vi "Tag Watchlist UI.vi"(6 "Shutdown Event":refnum<user-event>) -> ()   [LabVIEW 2020, in "Tag Watchlist.lvlib"]
doc: "Tag Watchlist window can view and modify any existing Tag.\n\nUse the Watchlist launcher to run this VI in your application."
uses:
  Tag Watchlist.lvlib
  Tag/Tag.lvclass
  Tag/Tag.lvclass/Tag.ctl
  Tag/Read Name.vi
  Tag/Read Type.vi
  Tag/Read Description.vi
  Tag/Read Units.vi
  Tag/Read Stale.vi
  Tag/Read Value.vi
  Tag/Read Timestamp.vi
  Core/Tag Lookup_By Name.vi
  <vilib>/Utility/Data Type/Get Type Information.vi
  <vilib>/JDP Science/JSONtext/Variant to JSON Text.vi
  Tag Engine.lvlib
panel:
  in  "Watchlist":i32(listbox)
  in  "Tag List":i32(listbox)
  in  "Filter":string
  # "Tag Engine Debug Watchlist Window"
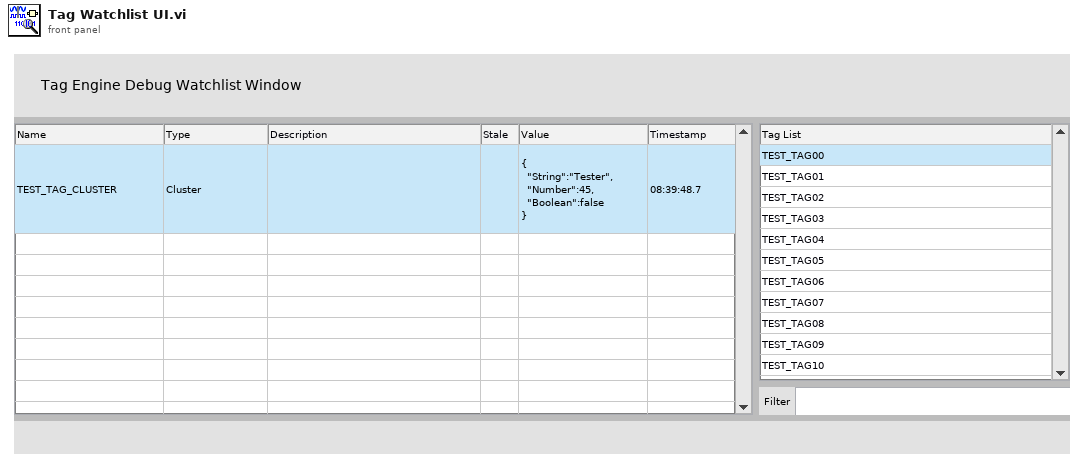
[diagram p1: front panel]
types:
  T1 = typedef "LVPoint32TypeDef.ctl" = cluster{"Horizontal":i32, "Vertical":i32}
  T2 = typedef "NI_Data Type.lvlib/Data Type.ctl" = enum8{"Invalid Type", "Void", "I8", "I16", "I32", "I64", "U8", "U16", "U32", "U64", "Single Float", "Double Float", "Extended Float", "Single Complex", "Double Complex", "Extended Complex", "Enum U8", "Enum U16", "Enum U32", "Enum U64", "Single Float With Unit", "Double Float With Unit", "Extended Float With Unit", "Single Complex with Unit", "Double Complex with Unit", "Extended Complex with Unit", "Boolean", "String", "Path", "Picture", "Tag", "Array", "Cluster", "Variant", "LV Variant", "Waveform", "Timestamp", "Digital Waveform", "Digital Data", "ExpressData", "Refnum", "External Data", "VI", "Poly VI", "LabVIEW Class Instance", "Fixed Point", "Set Collection", "Map Collection"}
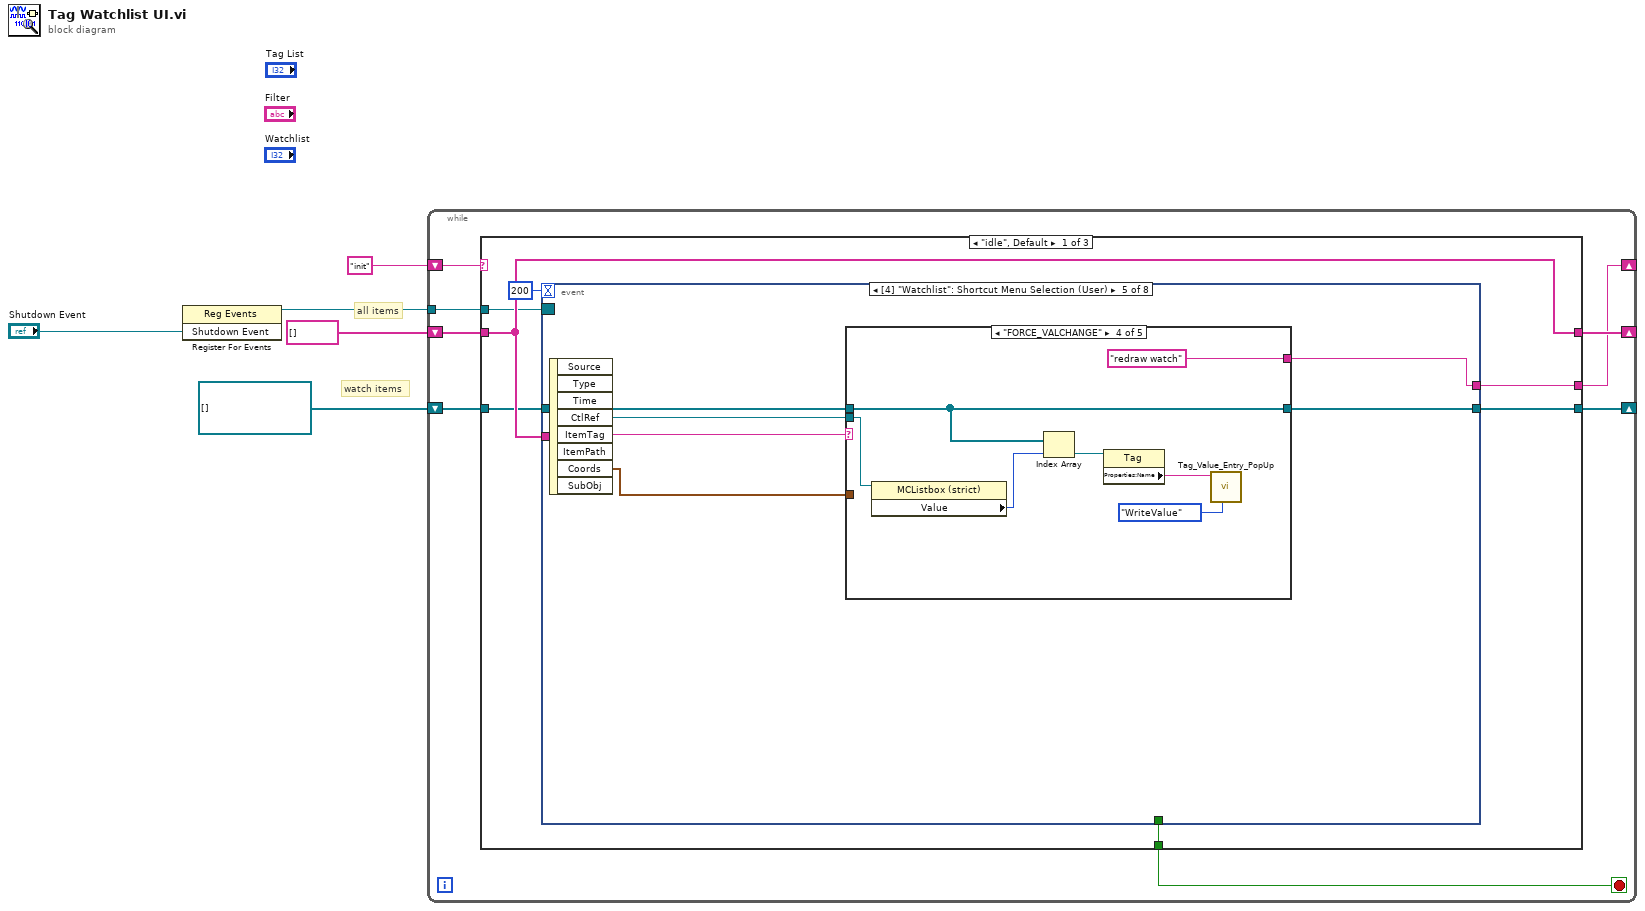
[diagram p0: block diagram]
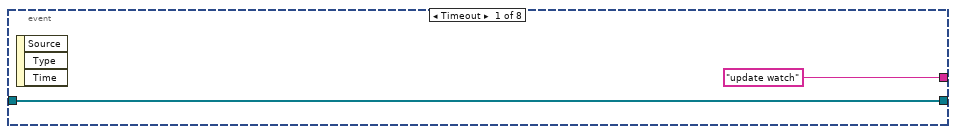
[diagram p2: hidden frame]
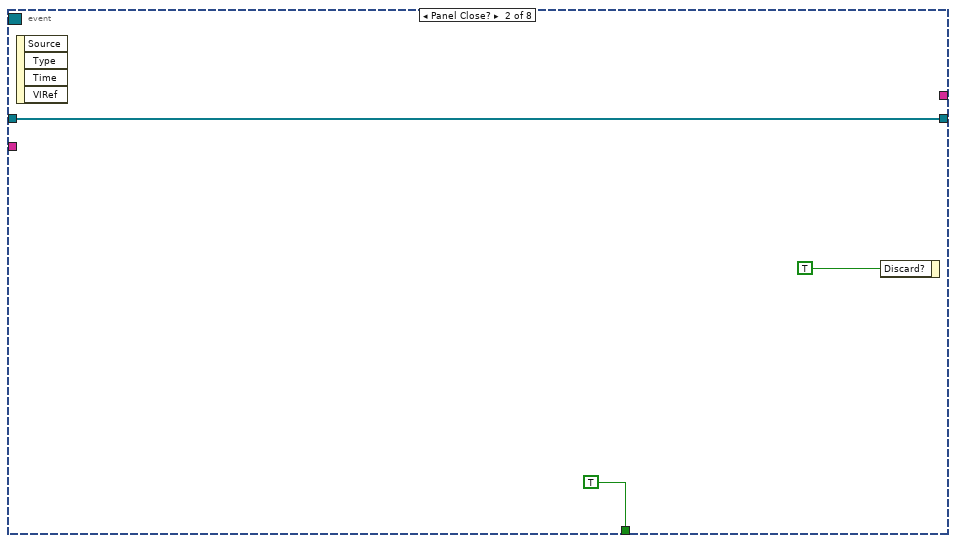
[diagram p3: hidden frame]
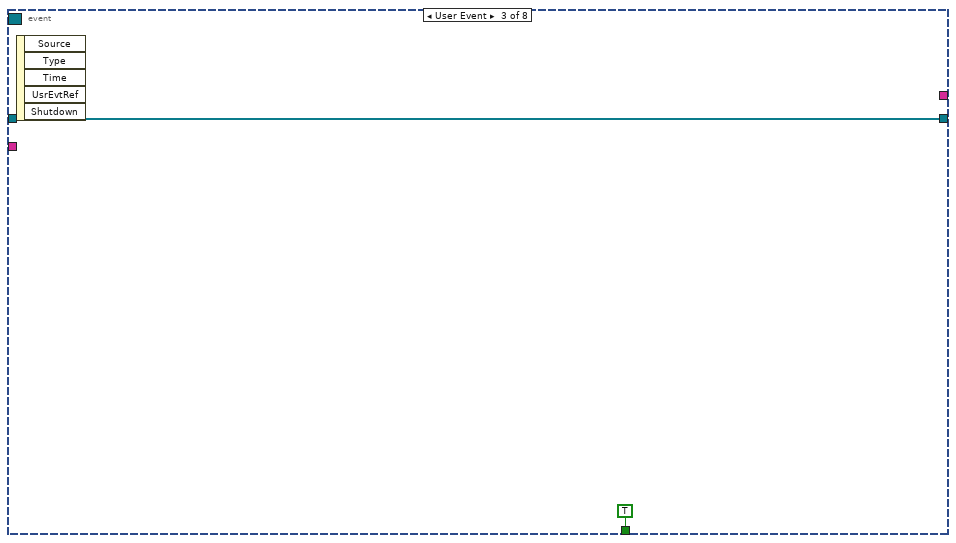
[diagram p4: hidden frame]
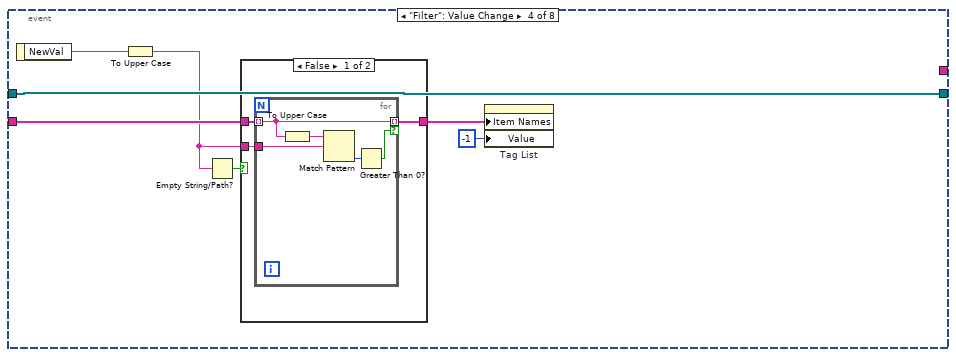
[diagram p5: hidden frame]
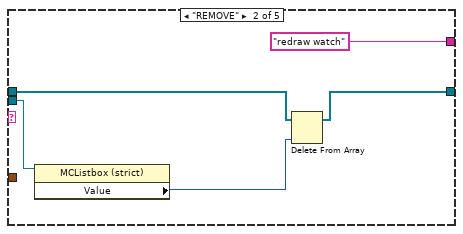
[diagram p8: hidden frame]
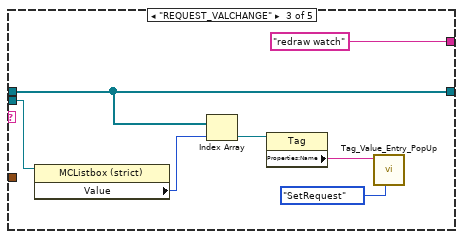
[diagram p9: hidden frame]
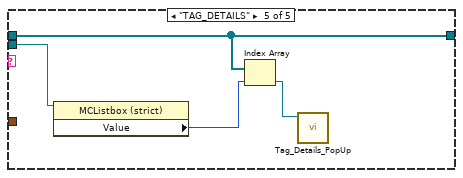
[diagram p10: hidden frame]
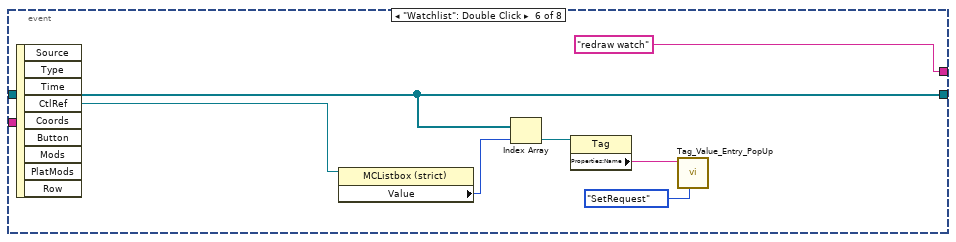
[diagram p11: hidden frame]
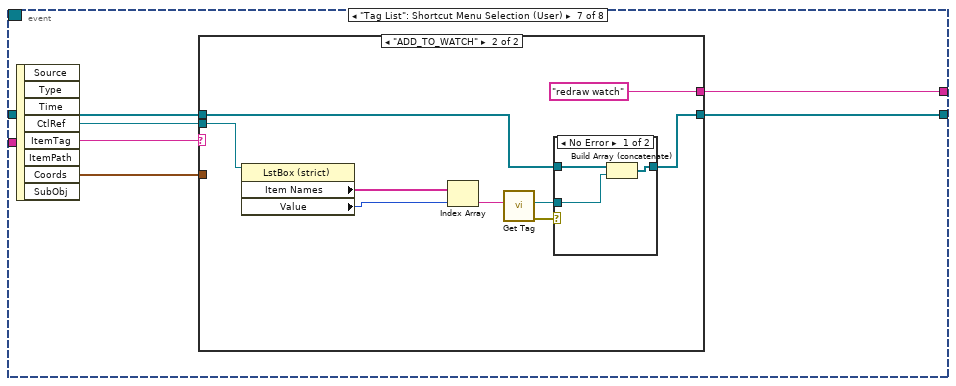
[diagram p12: hidden frame]
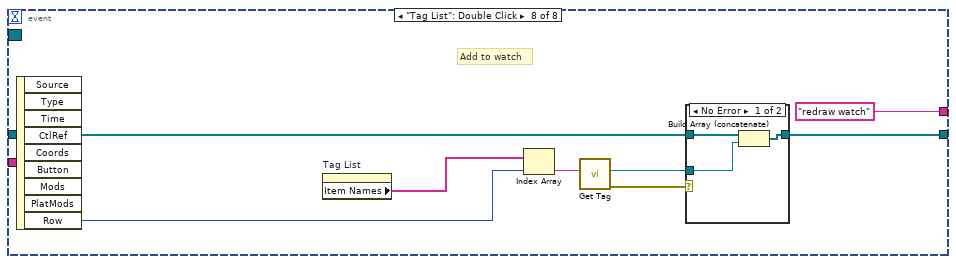
[diagram p15: hidden frame]
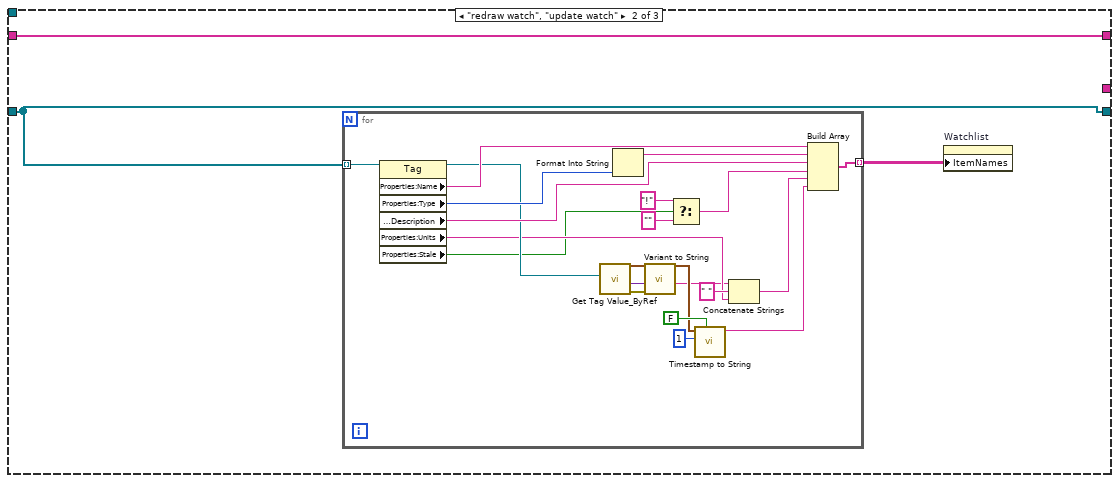
[diagram p17: hidden frame]
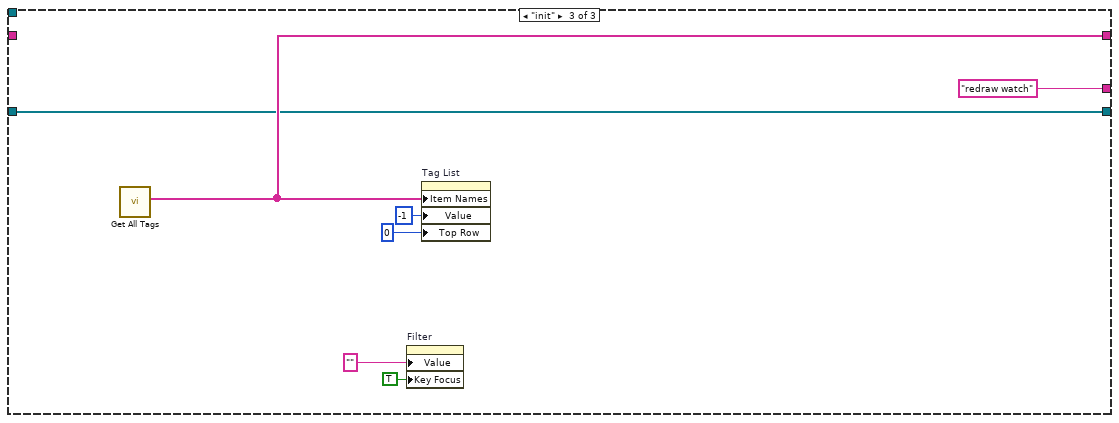
[diagram p18: hidden frame]
diagram:
  # "watch items"
  # "all items"
  n1 = register-events("Shutdown Event") -> (reference out=w2:refnum<event-registration>)  [unwired: 2 in, 1 out]
  n2 = while {
    shift-right: [w7] -> _
    shift-left: "init" -> [w13]
    shift-right: [w12] -> _
    shift-left: string[] [] ("Tag Names") -> [w11]
    shift-right: [w8] -> _
    shift-left: refnum<data-value>[] [] ("Item ref out") -> [w9]
    tunnel: w2 -> [w6]
    stop <- w10 stop-if-true
    n3 = case shown="\"idle\", Default" w13 {
      tunnel: [w19 w115 w143] -> w12
      tunnel: w11 -> [w19 w115 _]
      tunnel: [w20 _ _] -> w10
      tunnel: w9 -> [w18 w114 w142]
      tunnel: [w17 w114 w142] -> w8
      tunnel: [w15 _ "redraw watch"] -> w7
      tunnel: w6 -> [w14 _ _]
      frame "idle", Default {
        n4 = event shown="[4] \"Watchlist\": Shortcut Menu Selection (User)" {
          selector: w14 -> [_ _ _ _ _ _ _ _]
          dyn-events: _ -> [_ _ _ _ _ _ _ _]
          timeout: 200 -> [_ _ _ _ _ _ _ _]
          tunnel: [_ TRUE TRUE _ _ _ _ _] -> w20
          tunnel: w19 -> [_ _ _ w34 _ _ _ _]
          tunnel: w18 -> [w22 w23 w26 w31 w47 w80 w82 w108]
          tunnel: [w22 w23 w26 w31 w46 w80 w81 w107] -> w17
          tunnel: ["update watch" _ _ _ w45 "redraw watch" w85 "redraw watch"] -> w15
          event Timeout {
            n5 = event-data() -> ()  [unwired: 1 in, 3 out]
          }
          event Panel Close? {
            n6 = event-data() -> ()  [unwired: 1 in, 4 out]
            n7 = event-data("Discard?"=TRUE) -> ()  [unwired: 1 in, 1 out]
          }
          event User Event {
            n8 = event-data() -> ()  [unwired: 1 in, 5 out]
          }
          event "Filter": Value Change {
            n9 = event-data() -> ("NewVal"=w29:string)  [unwired: 1 in]
            n10 = To Upper Case(1:w29) -> (0:w28:string)
            n11 = Empty String/Path?(string/path=w28) -> (empty?=w30:bool)
            n12 = case shown="False" w30 {
              tunnel: w34 -> [w37 w43]
              tunnel: [w36 w43] -> w33
              tunnel: w28 -> [w35 _]
              frame False {
                n13 = for {
                  tunnel: w35 -> [w42]
                  tunnel: w37 -> [w39] mode=indexing
                  tunnel: [w39] -> w36 mode=indexing if=w40
                  n14 = To Upper Case(1:w39) -> (0:w38:string)
                  n15 = Match Pattern(string=w38, regular expression=w42) -> (offset past match=w41:i32)  [unwired: 1 in, 3 out]
                  n16 = Greater Than 0?(x=w41) -> (x > 0?=w40:bool)
                }
              }
              frame True {
              }
            }
            n17 = property on="Tag List" class="LstBox (strict)"("Item Names"=w33, "Value"=-1 ("Tag List")) -> ()  [unwired: 2 in, 2 out]
          }
          event "Watchlist": Shortcut Menu Selection (User) {
            n18 = event-data() -> ("CtlRef"=w44:refnum<vi>, "ItemTag"=w49:string, "Coords"=w48:T1)  [unwired: 1 in, 5 out]
            n19 = case shown="\"FORCE_VALCHANGE\"" w49 {
              tunnel: w48 -> [_ _ _ _ _]
              tunnel: w47 -> [w50 w55 w58 w65 w72]
              tunnel: [w50 w54 w58 w65 w72] -> w46
              tunnel: [_ "redraw watch" "redraw watch" "redraw watch" _] -> w45
              tunnel: w44 -> [_ w52 w61 w68 w73]
              frame Default {
              }
              frame "REMOVE" {
                n20 = property class="MCListbox (strict)"(reference=w52) -> ("Value"=w51:i32)  [unwired: 1 in, 2 out]
                n21 = Delete From Array(array=w55, index=w51) -> (array with subset deleted=w54:refnum<data-value>[])  [unwired: 1 in, 1 out]
              }
              frame "REQUEST_VALCHANGE" {
                n22 = property class="MCListbox (strict)"(reference=w61) -> ("Value"=w60:i32)  [unwired: 1 in, 2 out]
                n23 = Index Array(array=w58, index=w60) -> (element=w59:refnum<data-value>)
                n24 = property class="Tag"(reference=w59) -> ("Properties:Name"=w57:string)  [unwired: 1 in, 2 out]
                n25 = call "Tag_Value_Entry_PopUp.vi"("Write Type"=enum16{"SetRequest", "WriteValue"}."SetRequest", "Tag Name"=w57) -> ()  [unwired: 6 in, 4 out]
              }
              frame "FORCE_VALCHANGE" {
                n26 = property class="MCListbox (strict)"(reference=w68) -> ("Value"=w67:i32)  [unwired: 1 in, 2 out]
                n27 = Index Array(array=w65, index=w67) -> (element=w66:refnum<data-value>)
                n28 = property class="Tag"(reference=w66) -> ("Properties:Name"=w64:string)  [unwired: 1 in, 2 out]
                n29 = call "Tag_Value_Entry_PopUp.vi"("Write Type"=enum16{"SetRequest", "WriteValue"}."WriteValue", "Tag Name"=w64) -> ()  [unwired: 6 in, 4 out]
              }
              frame "TAG_DETAILS" {
                n30 = property class="MCListbox (strict)"(reference=w73) -> ("Value"=w71:i32)  [unwired: 1 in, 2 out]
                n31 = Index Array(array=w72, index=w71) -> (element=w70:refnum<data-value>)
                n32 = call "Tag_Details_PopUp.vi"("Tag Ref in"=w70) -> ()  [unwired: 10 in, 1 out]
              }
            }
          }
          event "Watchlist": Double Click {
            n33 = event-data() -> ("CtlRef"=w78:refnum<vi>)  [unwired: 1 in, 8 out]
            n34 = property class="MCListbox (strict)"(reference=w78) -> ("Value"=w77:i32)  [unwired: 1 in, 2 out]
            n35 = Index Array(array=w80, index=w77) -> (element=w76:refnum<data-value>)
            n36 = property class="Tag"(reference=w76) -> ("Properties:Name"=w75:string)  [unwired: 1 in, 2 out]
            n37 = call "Tag_Value_Entry_PopUp.vi"("Write Type"=enum16{"SetRequest", "WriteValue"}."SetRequest", "Tag Name"=w75) -> ()  [unwired: 6 in, 4 out]
          }
          event "Tag List": Shortcut Menu Selection (User) {
            n38 = event-data() -> ("CtlRef"=w84:refnum<vi>, "ItemTag"=w86:string, "Coords"=w83:T1)  [unwired: 1 in, 5 out]
            n39 = case shown="\"ADD_TO_WATCH\"" w86 {
              tunnel: [_ "redraw watch"] -> w85
              tunnel: w84 -> [_ w91]
              tunnel: w83 -> [_ _]
              tunnel: w82 -> [w87 w90]
              tunnel: [w87 w89] -> w81
              frame Default {
              }
              frame "ADD_TO_WATCH" {
                n40 = property on="Property Node" class="LstBox (strict)"(reference=w91) -> ("Item Names"=w95:string[], "Value"=w88:i32)  [unwired: 1 in, 2 out]
                n41 = Index Array(array=w95, index=w88) -> (element=w94:string)
                n42 = call "Get Tag.vi"("Name"=w94) -> ("error out"=w93:errorcluster, "Tag Ref out"=w92:refnum<data-value>)  [unwired: 8 in, 1 out]
                n43 = case shown="No Error" w93 {
                  tunnel: w90 -> [w99 w100]
                  tunnel: w92 -> [w98 _]
                  tunnel: [w97 w100] -> w89
                  frame No Error {
                    n44 = Build Array (concatenate)(w99, w98) -> (w97:refnum<data-value>[])
                  }
                  frame Error {
                  }
                }
              }
            }
          }
          event "Tag List": Double Click {
            # "Add to watch"
            n45 = event-data() -> ("Row"=w102:i32)  [unwired: 1 in, 8 out]
            n46 = property on="Tag List" class="LstBox (strict)"() -> ("Item Names"=w106:string[])  [unwired: 2 in, 2 out]
            n47 = Index Array(array=w106, index=w102) -> (element=w105:string)
            n48 = call "Get Tag.vi"("Name"=w105) -> ("error out"=w104:errorcluster, "Tag Ref out"=w103:refnum<data-value>)  [unwired: 8 in, 1 out]
            n49 = case shown="No Error" w104 {
              tunnel: w108 -> [w111 w112]
              tunnel: w103 -> [w110 _]
              tunnel: [w109 w112] -> w107
              frame No Error {
                n50 = Build Array (concatenate)(w111, w110) -> (w109:refnum<data-value>[])
              }
              frame Error {
              }
            }
          }
        }
      }
      frame "redraw watch", "update watch" {
        n51 = for {
          tunnel: w114 -> [w136] mode=indexing
          tunnel: [w128] -> w113 mode=indexing
          n52 = property class="Tag"(reference=w136) -> (reference out=w127:refnum<data-value>, "Properties:Name"=w134:string, "Properties:Type"=w135:T2, "Properties:Description"=w132:string, "Properties:Units"=w124:string, "Properties:Stale"=w122:bool)  [unwired: 1 in, 1 out]
          n53 = call "Get Tag Value_ByRef.vi"("Tag Ref in"=w127) -> ("error out"=w118:errorcluster, "Value"=w117:variant, "Timestamp"=w126:timestamp)  [unwired: 7 in, 1 out]
          n54 = Format Into String(w135) -> (resulting string=w133:string)  [unwired: 3 in, 1 out]
          n55 = call "Variant to String.vi"("error in"=w118, "Variant Value"=w117) -> ("String Value"=w116:string)  [unwired: 8 in, 1 out]
          n56 = Select(t="!", s=w122, f="") -> (s? t:f=w119:string)
          n57 = call "Timestamp to String.vi"("Include Date? (T)"=FALSE, "Precision (0)"=u8 1, "time stamp"=w126) -> ("date/time string"=w129:string)  [unwired: 8 in]
          n58 = Concatenate Strings(w116, " " ("string"), w124) -> (w123:string)
          n59 = Build Array(w134, w133, w132, w119, w123, w129) -> (w128:string[])
        }
        n60 = property on="Watchlist" class="MCListbox (strict)"("ItemNames"=w113) -> ()  [unwired: 2 in, 2 out]
      }
      frame "init" {
        n61 = call "Get All Tags.vi"() -> ("Tag Names"=w143:string[])  [unwired: 9 in, 2 out]
        n62 = property on="Filter" class="Str"("Value"="" ("Filter"), "Key Focus"=TRUE) -> ()  [unwired: 2 in, 2 out]
        n63 = property on="Tag List" class="LstBox (strict)"("Item Names"=w143, "Value"=-1 ("Tag List"), "Top Row"=0) -> ()  [unwired: 2 in, 2 out]
      }
    }
  }
